vi "TC_S_VtoC.vi"(11 "Thermocouple Voltage":dbl caption="热电偶电压" format="%0.6f") -> (3 "T(c)":dbl format="%#_16f")   [LabVIEW 2012]
doc: "功能：\n\nS型热电偶电压转换为摄氏度。\n\ncsxcs_366创建。"
uses:
  <vilib>/Analysis/polynomials.llb/Scalar Polynomial Evaluation (DBL).vi
  <vilib>/Analysis/NI_AALPro.lvlib
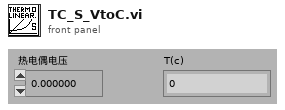
[diagram p1: front panel]
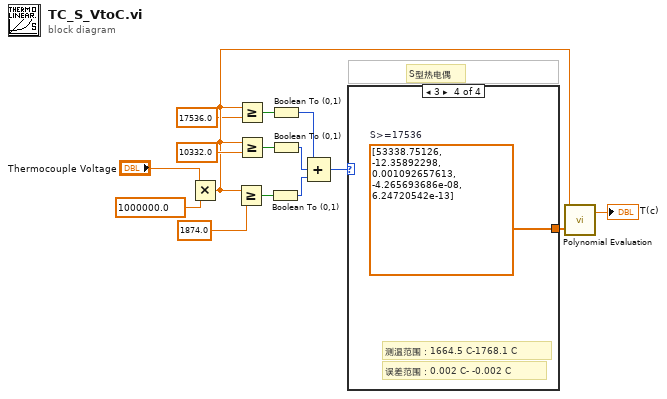
[diagram p0: block diagram]
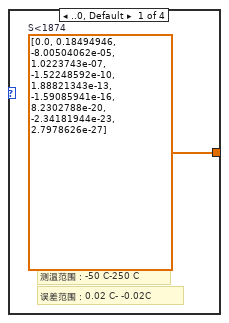
[diagram p2: hidden frame]
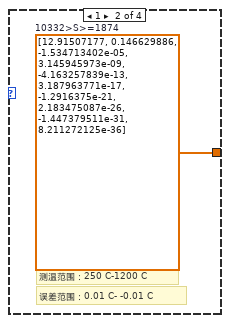
[diagram p3: hidden frame]
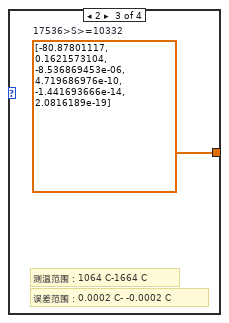
[diagram p4: hidden frame]
diagram:
  # "S型热电偶"
  n1 = Multiply(x="Thermocouple Voltage", y=1000000.0) -> (x*y=w3:dbl)
  n2 = Greater Or Equal?(x=w3, y=1874.0) -> (x >= y?=w9:bool)
  n3 = Greater Or Equal?(x=w3, y=17536.0) -> (x >= y?=w5:bool)
  n4 = Greater Or Equal?(x=w3, y=10332.0) -> (x >= y?=w10:bool)
  n5 = Boolean To (0,1)(Boolean=w9) -> (0, 1=w8:i16)
  n6 = Boolean To (0,1)(Boolean=w5) -> (0, 1=w4:i16)
  n7 = Boolean To (0,1)(Boolean=w10) -> (0, 1=w7:i16)
  n8 = Compound Arithmetic op=ADD(w4, w7, w8) -> (w6:i16)
  n9 = case shown="3" w6 {
    tunnel: [w16 w17 w18 w19] -> w1
    frame ..0, Default {
      w16 = dbl[] [0.0, 0.18494946, -8.00504062e-05, 1.0223743e-07, -1.52248592e-10, 1.88821343e-13, -1.59085941e-16, 8.2302788e-20, -2.34181944e-23, 2.7978626e-27]  # S<1874
      # "误差范围：0.02 C- -0.02C"
      # "测温范围：-50 C-250 C"
    }
    frame 1 {
      w17 = dbl[] [12.91507177, 0.146629886, -1.534713402e-05, 3.145945973e-09, -4.163257839e-13, 3.187963771e-17, -1.2916375e-21, 2.183475087e-26, -1.447379511e-31, 8.211272125e-36]  # 10332>S>=1874
      # "误差范围：0.01 C- -0.01 C"
      # "测温范围：250 C-1200 C"
    }
    frame 2 {
      w18 = dbl[] [-80.87801117, 0.1621573104, -8.536869453e-06, 4.719686976e-10, -1.441693666e-14, 2.0816189e-19]  # 17536>S>=10332
      # "误差范围：0.0002 C- -0.0002 C"
      # "测温范围：1064 C-1664 C"
    }
    frame 3 {
      w19 = dbl[] [53338.75126, -12.35892298, 0.001092657613, -4.265693686e-08, 6.24720542e-13]  # S>=17536
      # "误差范围：0.002 C- -0.002 C"
      # "测温范围：1664.5 C-1768.1 C"
    }
  }
  n10 = call-poly <vilib>:"Polynomial Evaluation.vi"("P(x)"=w1, "a"=w3) -> ("P(a)"=→"T(c)":dbl)  [unwired: 1 out]
